vi "PIManager.vi"(3 "error in (no error)":errorcluster caption="错误输入（无错误）", 4 "Input":T1, 5 "ref in":string[](array[string])) -> (0 "error out":errorcluster caption="错误输出", 1 "Output":T1, 2 "ref out":string[](array[string]))   [LabVIEW 2012]
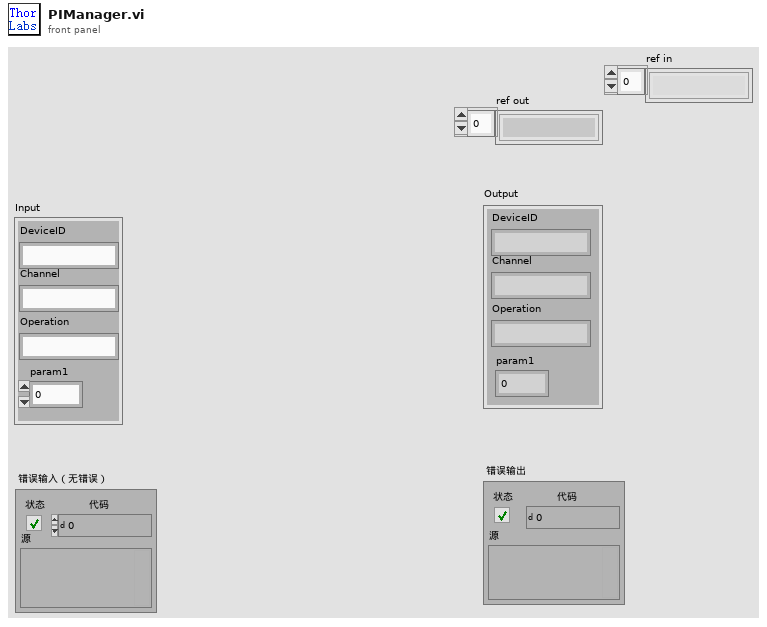
[diagram p1: front panel]
types:
  T1 = cluster{"DeviceID":string, "Channel":string, "param1":dbl, "Operation":string}
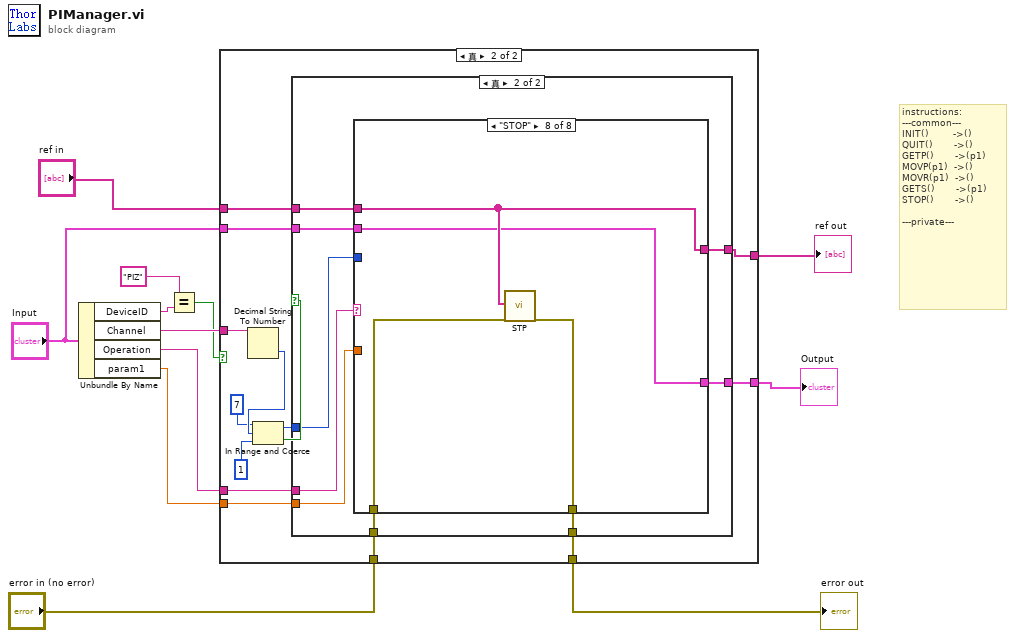
[diagram p0: block diagram]
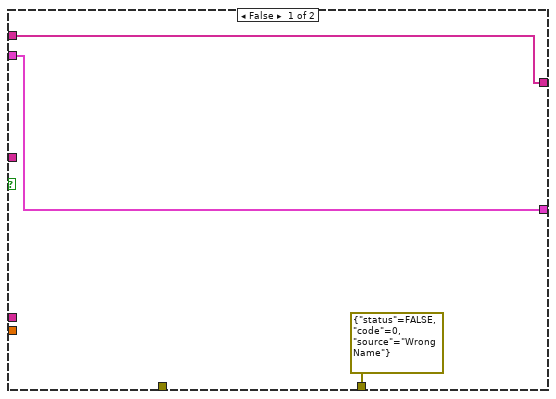
[diagram p2: hidden frame]
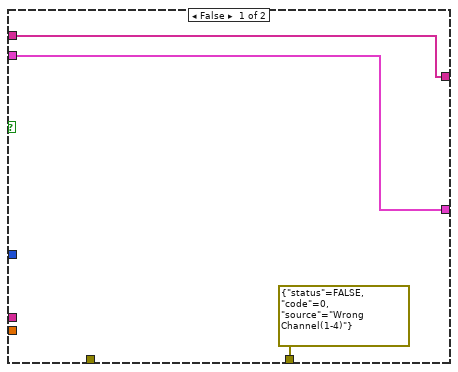
[diagram p3: hidden frame]
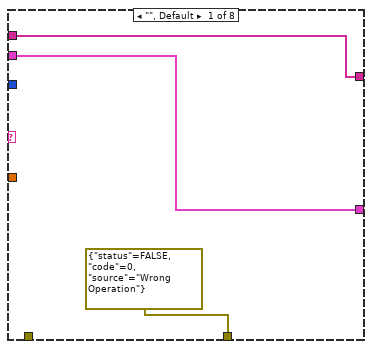
[diagram p4: hidden frame]
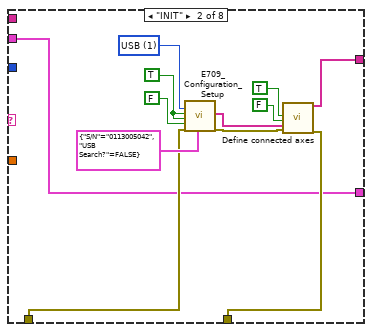
[diagram p5: hidden frame]
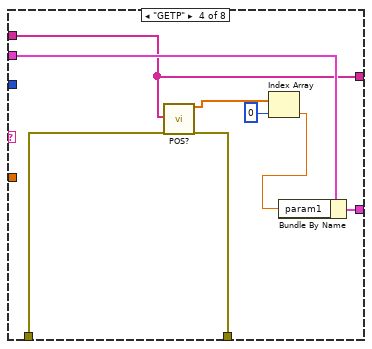
[diagram p7: hidden frame]
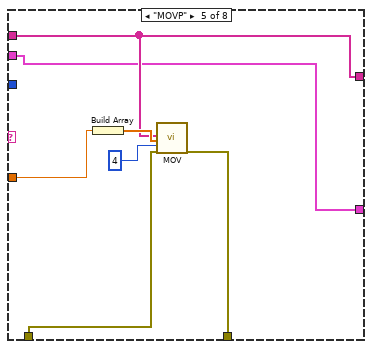
[diagram p8: hidden frame]
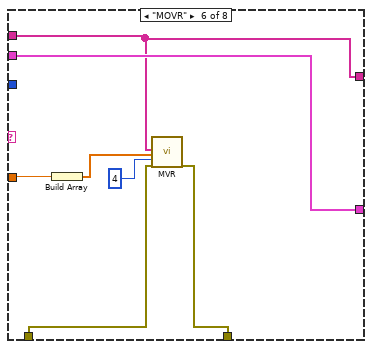
[diagram p9: hidden frame]
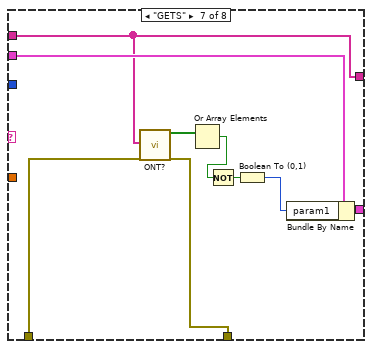
[diagram p10: hidden frame]
diagram:
  # "instructions:\n---common---\nINIT()        ->()\nQUIT()       ->()\nGETP()       ->(p1)\nMOVP(p1)  ->()\nMOVR(p1)  ->()\nGETS()       ->(p1)\nSTOP()       ->()\n\n---private---"
  n1 = Unbundle By Name("Input") -> ("DeviceID"=w12:string, "Channel"=w10:string, "Operation"=w9:string, "param1"=w8:dbl)
  n2 = Equal?(x="PIZ", y=w12) -> (x = y?=w3:bool)
  n3 = case shown="真" w3 {
    tunnel: w10 -> [_ w29]
    tunnel: w9 -> [_ w23]
    tunnel: w8 -> [_ w22]
    tunnel: "error in (no error)" -> [_ w21]
    tunnel: [errorcluster {"status"=FALSE, "code"=0, "source"="Wrong Name"} ("error out") w20] -> w6
    tunnel: [w15 w19] -> w5
    tunnel: "ref in" -> [w13 w18]
    tunnel: "Input" -> [w15 w17]
    tunnel: [w13 w16] -> w2
    frame False {
    }
    frame True {
      n4 = Decimal String To Number(string=w29) -> (number=w28:i32)  [unwired: 2 in, 1 out]
      n5 = In Range and Coerce(upper limit=7 ("上限"), x=w28, lower limit=1 ("下限")) -> (coerced(x)=w24:i32, In Range?=w25:bool)
      n6 = case shown="真" w25 {
        tunnel: w24 -> [_ w33]
        tunnel: w23 -> [_ w41]
        tunnel: w22 -> [_ w40]
        tunnel: w21 -> [_ w39]
        tunnel: [errorcluster {"status"=FALSE, "code"=0, "source"="Wrong Channel(1-4)"} ("error out") w38] -> w20
        tunnel: [w32 w37] -> w19
        tunnel: w18 -> [w30 w34]
        tunnel: w17 -> [w32 w36]
        tunnel: [w30 w35] -> w16
        frame False {
        }
        frame True {
          n7 = case shown="\"STOP\"" w41 {
            tunnel: w33 -> [_ _ _ _ _ _ _ _]
            tunnel: w40 -> [_ _ _ _ w73 w81 _ _]
            tunnel: w39 -> [_ w47 w59 w67 w71 w78 w90 w94]
            tunnel: [errorcluster {"status"=FALSE, "code"=0, "source"="Wrong Operation"} ("error out") w48 w59 w66 w70 w77 w88 w93] -> w38
            tunnel: [w44 w45 w57 w61 w68 w76 w85 w91] -> w37
            tunnel: w34 -> [w42 _ w58 w62 w69 w75 w82 w92]
            tunnel: w36 -> [w44 w45 w57 w63 w68 w76 w84 w91]
            tunnel: [w42 w46 w58 w62 w69 w75 w82 w92] -> w35
            frame "", Default {
            }
            frame "INIT" {
              w53 = TRUE ("Connected?")
              w56 = u16 1 items=["RS232", "USB"] ("Interface")
              n8 = call "E709_Configuration_Setup.vi"("Interface"=w56, "Connected?"=w53, "Change servo status to ON?"=w53, "Perform autozero?"=FALSE, "error in"=w47, "USB settings"=cluster{"S/N":string, "USB Search?":bool} {"S/N"="0113005042", "USB Search?"=FALSE}) -> ("Conn. \nAxis"=w50:string[], "error out"=w49:errorcluster)  [unwired: 8 in, 4 out]
              n9 = call "Define connected axes.vi"("Read from\ncontroller?"=TRUE ("Read from\ncontroller?"), "Invert\norder?"=FALSE ("Invert\norder?"), "Conn. axes"=w50, "error in"=w49) -> ("Conn. Axes out"=w46:string[], "error out"=w48:errorcluster)  [unwired: 14 in]
            }
            frame "QUIT" {
            }
            frame "GETP" {
              n10 = call "POS?.vi"("Axes to query"=w62, "error in"=w67) -> ("Position"=w64:dbl[], "error out"=w66:errorcluster)  [unwired: 16 in]
              n11 = Index Array(array=w64, index=0 ("索引")) -> (element=w60:dbl)
              n12 = Bundle By Name(cluster=w63, "param1"=w60) -> (w61:T1)
            }
            frame "MOVP" {
              n13 = Build Array(w73) -> (w74:dbl[])
              n14 = call "MOV.vi"("Axes to move"=w69, "Position values"=w74, "No.of digits"=i16 4, "error in"=w71) -> ("error out"=w70:errorcluster)  [unwired: 15 in]
            }
            frame "MOVR" {
              n15 = Build Array(w81) -> (w80:dbl[])
              n16 = call "MVR.vi"("Axes to move"=w75, "Position values"=w80, "No.of digits"=i16 4, "error in"=w78) -> ("error out"=w77:errorcluster)  [unwired: 15 in]
            }
            frame "GETS" {
              n17 = call "ONT?.vi"("Axes to query"=w82, "error in"=w90) -> ("Axis on target?"=w89:bool[], "error out"=w88:errorcluster)  [unwired: 16 in]
              n18 = Or Array Elements(Boolean array=w89) -> (logical OR=w87:bool)
              n19 = Not(x=w87) -> (.not. x?=w86:bool)
              n20 = Boolean To (0,1)(Boolean=w86) -> (0, 1=w83:i16)
              n21 = Bundle By Name(cluster=w84, "param1"=w83) -> (w85:T1)
            }
            frame "STOP" {
              n22 = call "STP.vi"("Affected axes?"=w92, "error in"=w94) -> ("error out"=w93:errorcluster)  [unwired: 17 in]
            }
          }
        }
      }
    }
  }
  "Output" <- w5
  "error out" <- w6
  "ref out" <- w2
